vi "niDTS Calibration Cal Execute RF Test Get Documentation.vi"(0 "Template Tx Test Handle in":T2, 11 "error in (no error)":errorcluster) -> (4 "Template Tx Test Handle out":T2, 8 "Documentation":T1, 15 "error out":errorcluster)   [LabVIEW 2014, in "niDTS Utilities.lvlib"]
uses:
  niDTS Utilities.lvlib
  Includes/niDTS Calibration Cal Execute RF Test INC Handle.ctl
  Objects/BASE_class/niDTS Calibration Cal Execute RF Test.lvclass
  Framework/Test/Includes/niDTS Test INC Documentation.ctl
  Framework/niDTS Framework.lvlib
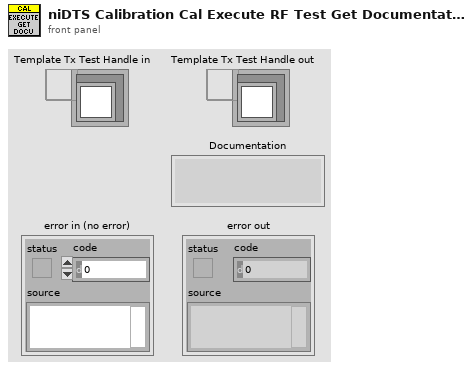
[diagram p1: front panel]
types:
  T1 = typedef "niDTS Framework.lvlib/niDTS Test INC Documentation.ctl" = string
  T2 = typedef "niDTS Utilities.lvlib/niDTS Calibration Cal Execute RF Test INC Handle.ctl" = refnum<data-value>
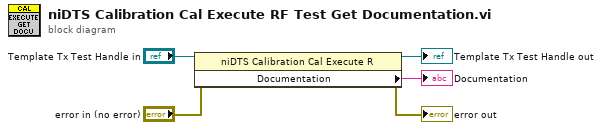
[diagram p0: block diagram]
diagram:
  n1 = property class="niDTS Calibration Cal Execute R"(reference="Template Tx Test Handle in", error in="error in (no error)") -> (reference out=→"Template Tx Test Handle out":T2, error out=→"error out":errorcluster, "Documentation"=→"Documentation":T1)
